vi "Read JSON message 1.vi"(8 "error in (no error)":errorcluster, 11 "Channel in":refnum<class "Channel.lvclass">) -> (0 "error out":errorcluster, 2 "JSON message":T1, 3 "Channel out":refnum<class "Channel.lvclass">)   [LabVIEW 2018, in "Channel.lvclass"]
uses:
  Channel.lvclass
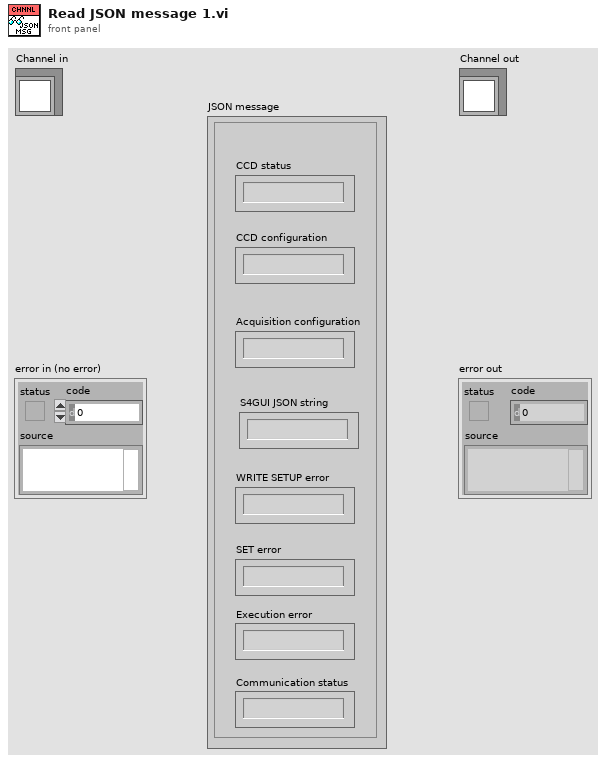
[diagram p1: front panel]
types:
  T1 = cluster{"CCD status":string, "CCD configuration":string, "Acquisition configuration":string, "S4GUI JSON string":string, "WRITE SETUP error":string, "Execution error":string, "SET error":string, "Communication status":string}
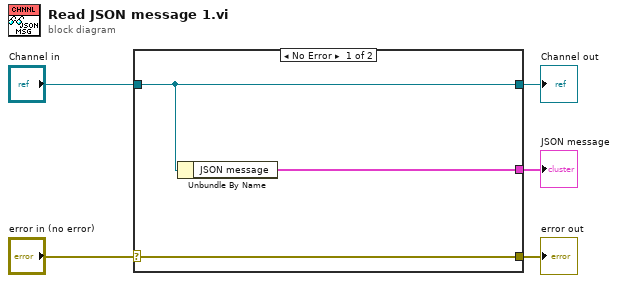
[diagram p0: block diagram]
diagram:
  n1 = case shown="No Error" "error in (no error)" {
    selector: "error in (no error)" -> [w8 w9]
    tunnel: [w8 w9] -> w4
    tunnel: [w7 w10] -> w2
    tunnel: "Channel in" -> [w7 w10]
    tunnel: [w6 _] -> w1
    frame No Error {
      n2 = Unbundle By Name(w7) -> ("JSON message"=w6:T1)
    }
    frame Error {
    }
  }
  "error out" <- w4
  "Channel out" <- w2
  "JSON message" <- w1
